vi "Normalized to Encoder Velocity.vi"(8 "Enum":enum16{"Vantage", "Mule", "Linda/Sophie"}(ring), 11 "ft/s":dbl) -> (3 "Output":dbl)   [LabVIEW 2018]
doc: "Converting from ft/s to Rev/min (for sparks) or ticks/100ms (for Talons)"
panel:
  in  "y":dbl=0.85 format="%#_13g"
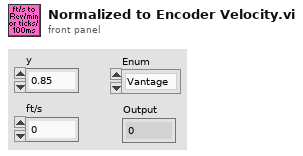
[diagram p1: front panel]
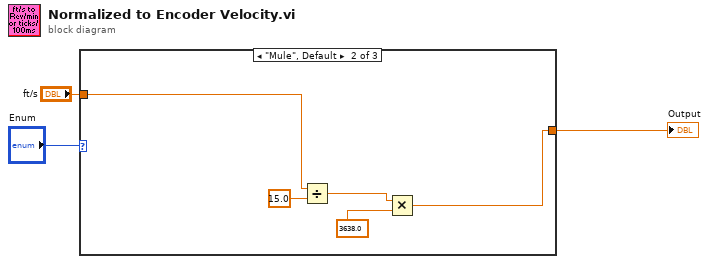
[diagram p0: block diagram]
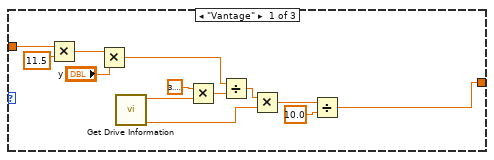
[diagram p2: hidden frame]
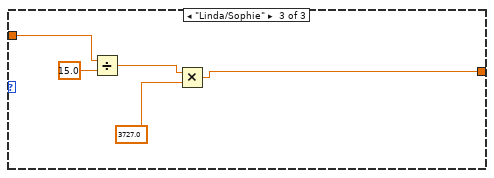
[diagram p3: hidden frame]
diagram:
  n1 = case shown="\"Mule\", Default" "Enum" {
    tunnel: "ft/s" -> [w16 w19 w26]
    tunnel: [w4 w18 w22] -> w1
    frame "Vantage" {
      n2 = Multiply(x=w16, y=11.5) -> (x*y=w7:dbl)
      n3 = Multiply(x=w7, y="y") -> (x*y=w5:dbl)
      n4 = call "Get Drive Information.vi"() -> ("Ticks/Revolution"=w8:dbl, "Wheel Diameter"=w9:dbl)  [unwired: 10 in]
      n5 = Multiply(x=3.141592653589793, y=w9) -> (x*y=w13:dbl)
      n6 = Divide(x=w5, y=w13) -> (x/y=w12:dbl)
      n7 = Multiply(x=w12, y=w8) -> (x*y=w11:dbl)
      n8 = Divide(x=w11, y=10.0) -> (x/y=w4:dbl)
    }
    frame "Mule", Default {
      n9 = Divide(x=w19, y=15.0) -> (x/y=w20:dbl)
      n10 = Multiply(x=w20, y=3638.0 ("y 2")) -> (x*y=w18:dbl)
    }
    frame "Linda/Sophie" {
      n11 = Divide(x=w26, y=15.0) -> (x/y=w24:dbl)
      n12 = Multiply(x=w24, y=3727.0 ("Scaling")) -> (x*y=w22:dbl)
    }
  }
  "Output" <- w1
